vi "Tab Control Example.vi"() -> ()   [LabVIEW 2020]
doc: "This VI is not used in the final structure, it is simply a demonstration of the basic structure of the software. The basics are as follows:\n- Create a connection with the machine's controller\n- Send it a series of commands depending on which tab the user selects\n- Close the connection with the machine's controller"
uses:
  <instrlib>/Arcus Ethernet Driver 1.0.0/ArcusEthernetComm/classes/Controller/_Controller.lvclass
panel:
  in  "Tab Control":T1(tab)
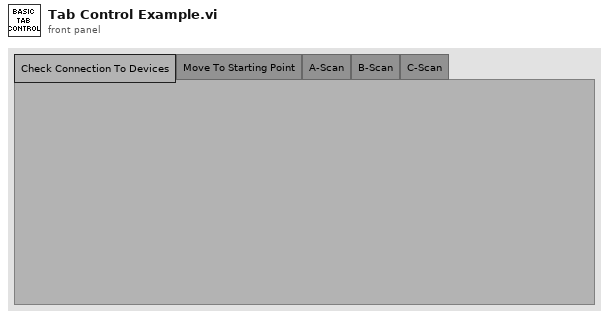
[diagram p1: front panel]
types:
  T1 = enum32{"Check Connection To Devices", "Move To Starting Point", "A-Scan", "B-Scan", "C-Scan"}
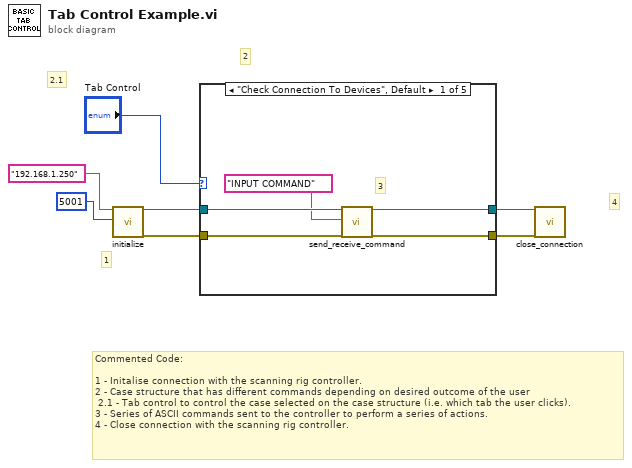
[diagram p0: block diagram]
diagram:
  # "2"
  # "4"
  # "2.1"
  # "1"
  # "Commented Code:\n\n1 - Initalise connection with the scanning rig controller.\n2 - Case structure that has different commands depending on desired outcome of the user\n 2.1 - Tab control to control the case selected on the case structure (i.e. which tab the user clicks).\n3 - Series of ASCII commands sent to the controller to perform a series of actions.\n4 - Close connection with the scanning rig controller."
  n1 = call <instrlib>:"initialize.vi"("ip_address (in)"="192.168.1.250", "dev_port(def=5001)"=u16 5001) -> ("reference (out)"=w4:refnum<class "_Controller.lvclass">, "error out"=w2:errorcluster)  [unwired: 16 in]
  n2 = case shown="\"Check Connection To Devices\", Default" "Tab Control" {
    tunnel: w4 -> [w11 _ _ _ _]
    tunnel: [w12 _ _ _ _] -> w3
    tunnel: w2 -> [w10 _ _ _ _]
    tunnel: [w9 _ _ _ _] -> w1
    frame "Check Connection To Devices", Default {
      # "3"
      n3 = call <instrlib>:"send_receive_command.vi"("reference (in)"=w11, "ASCII Command (in)"="INPUT COMMAND", "error in (no error)"=w10) -> ("reference (out)"=w12:refnum<class "_Controller.lvclass">, "error out"=w9:errorcluster)  [unwired: 12 in, 3 out]
    }
    frame "Move To Starting Point" {
    }
    frame "A-Scan" {
    }
    frame "B-Scan" {
    }
    frame "C-Scan" {
    }
  }
  n4 = call <instrlib>:"close_connection.vi"("reference (in)"=w3, "error in (no error)"=w1) -> ()  [unwired: 16 in, 2 out]
